vi "Index.vi"(8 "error in (no error)":errorcluster, 10 "Index":i32, 11 "Enum Array in":refnum<class "Enum Array.lvclass">) -> (0 "error out":errorcluster, 3 "Indexed element":refnum<class "Generic Data.lvclass">)   [LabVIEW 2020, in "Data.lvlib" / "Enum Array.lvclass"]
doc: "Index an element from 'Generic Data in'.\nThis implementation returns a generic Enum class with the indexed Enum."
uses:
  Enum Array.lvclass
  Generic Data.lvclass
  Enum Array.lvclass/Enum Array.ctl
  Enum/Enum.lvclass/Enum.ctl
  Enum/Enum.lvclass
  C:/Users/Henri/OneDrive/LabVIEW/Framework/Data/Generic Data/Generic Data.lvclass
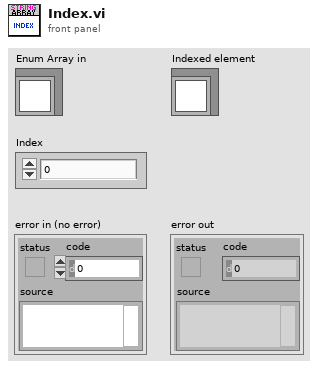
[diagram p1: front panel]
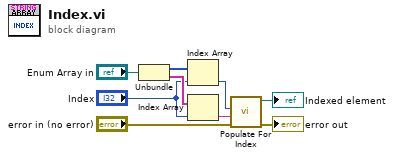
[diagram p0: block diagram]
diagram:
  n1 = Unbundle("Enum Array in") -> (w8:u32[], w7:string[])
  n2 = Index Array(array=w8, index="Index") -> (element=w5:u32)
  n3 = Index Array(array=w7, index="Index") -> (element=w4:string)
  n4 = call "Populate For Index.vi"("error in (no error)"="error in (no error)", "Enum Alias"=w4, "Enum Index"=w5) -> ("error out"=→"error out":errorcluster, "Enum out"=→"Indexed element":refnum<class "Enum.lvclass">)  [unwired: 7 in]
